vi "PC Host Demo.vi"() -> ()   [LabVIEW 2015]
doc: "该模板用于创建生产者／消费者模式的应用程序，以事件驱动的方式，生成队列中的项。如需通过响应事件实现代码的异步执行，同时不影响用户界面的响应速度，可考虑用该模式替代用户界面事件处理器模式。"
panel:
  in  "Galvo Waveform file path":path=path "C:/Users/LOCI/Documents/MATLAB/ScanImage/scanner signal/xx.txt"
  out "数据（可为任意类型）":string
  in  "Enqueue Element":bool caption="元素入队列"
  in  "stop":bool caption="停止"
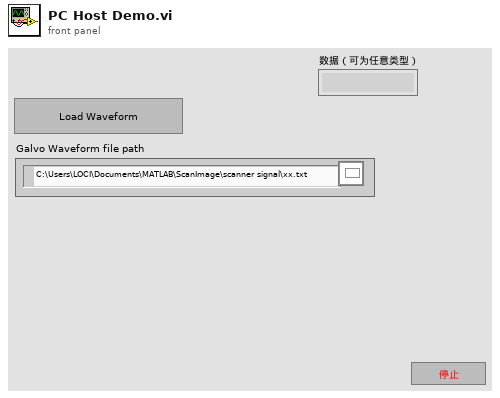
[diagram p1: front panel]
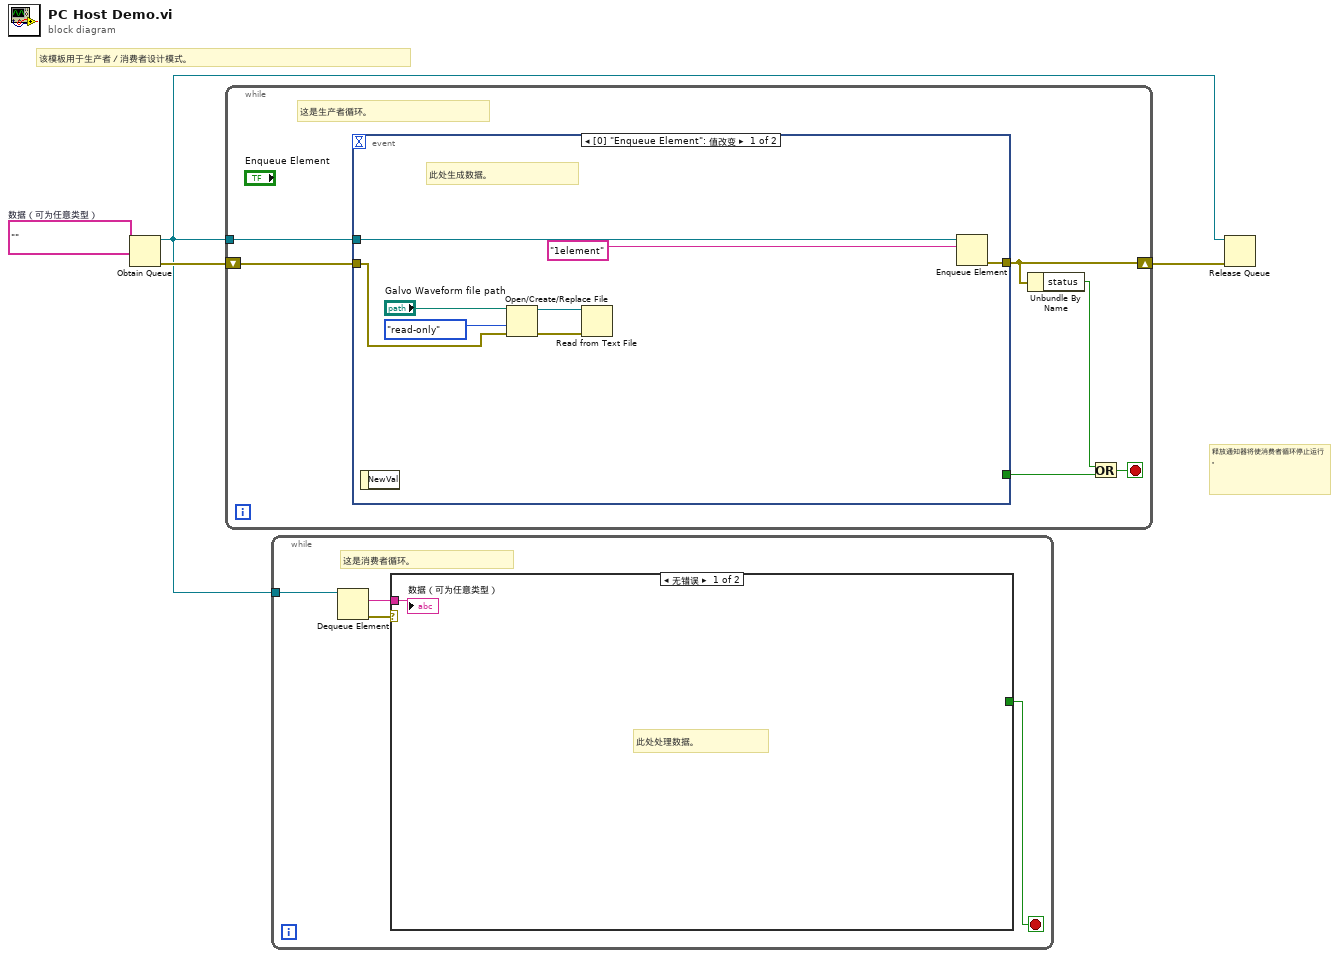
[diagram p0: block diagram]
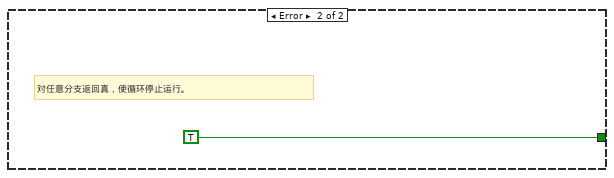
[diagram p2: hidden frame]
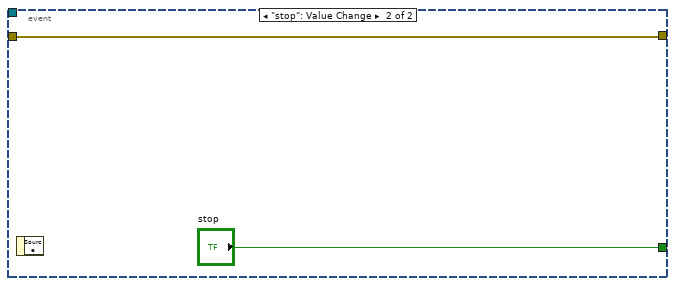
[diagram p3: hidden frame]
diagram:
  w2 = ""  # 数据（可为任意类型）
  # "释放通知器将使消费者循环停止运行。"
  # "该模板用于生产者／消费者设计模式。"
  n1 = Obtain Queue(element data type=w2) -> (queue out=w1:refnum<queue>, error out=w4:errorcluster)  [unwired: 4 in, 1 out]
  n2 = while {
    shift-right: [w6] -> w3
    shift-left: w4 -> [w9]
    tunnel: w1 -> [w10]
    stop <- w7 stop-if-true
    # "这是生产者循环。"
    n3 = event shown="[0] \"Enqueue Element\": 值改变" {
      selector: _ -> [_ _]
      dyn-events: _ -> [_ _]
      timeout: _ -> [_ _]
      tunnel: w10 -> [w18 _]
      tunnel: w9 -> [w13 w19]
      tunnel: [w17 w19] -> w6
      tunnel: [_ "stop"] -> w8
      event "Enqueue Element": Value Change {
        # "此处生成数据。"
        n4 = event-data() -> ()  [unwired: 1 in, 1 out]
        n5 = Open/Create/Replace File(file path (use dialog)="Galvo Waveform file path", error in=w13, access (0:read/write)=enum16{"read/write", "read-only", "write-only"}."read-only" ("权限(0:read/write)")) -> (refnum out=w12:refnum<file>, error out=w11:errorcluster)  [unwired: 3 in, 1 out]
        n6 = Read from Text File(file (use dialog)=w12, error in=w11) -> ()  [unwired: 2 in, 4 out]
        n7 = Enqueue Element(queue=w18, element="1element") -> (error out=w17:errorcluster)  [unwired: 2 in, 2 out]
      }
      event "stop": Value Change {
        n8 = event-data() -> ()  [unwired: 1 in, 1 out]
      }
    }
    n9 = Unbundle By Name(w6) -> ("status"=w5:bool)
    n10 = Or(x=w5, y=w8) -> (x .or. y?=w7:bool)
  }
  n11 = while {
    tunnel: w1 -> [w24]
    stop <- w21 stop-if-true
    # "这是消费者循环。"
    n12 = Dequeue Element(queue=w24) -> (element=w22:string, error out=w23:errorcluster)  [unwired: 2 in, 2 out]
    n13 = case shown="无错误" w23 {
      tunnel: w22 -> [w25 _]
      tunnel: [_ TRUE] -> w21
      frame No Error {
        # "此处处理数据。"
        "数据（可为任意类型）" <- w25
      }
      frame Error {
        # "对任意分支返回真，使循环停止运行。"
      }
    }
  }
  n14 = Release Queue(queue=w1, error in (no error)=w3) -> ()  [unwired: 1 in, 3 out]
